vi "InnerCallbackOnWriteTree.vi"(8 "error in":errorcluster, 10 "node (for type)":refnum<class "Engine Parent Editor Node.lvclass">, 11 "node reference":refnum<data-value>) -> (0 "error out":errorcluster)   [LabVIEW 2013, in "PL Framework Configuration Tool.lvlib" / "Engine Parent Editor Node.lvclass"]
uses:
  Engine Parent Editor Node.lvclass
  <vilib>/NI/Configuration Framework/Node/NISE_CEF_Node.lvclass
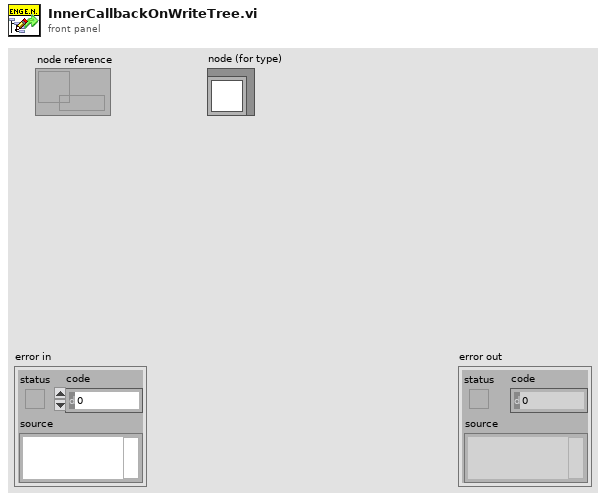
[diagram p1: front panel]
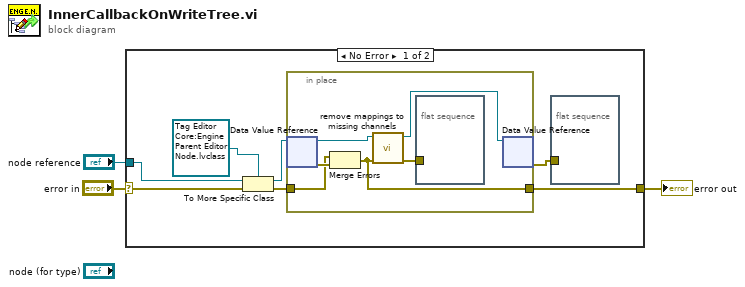
[diagram p0: block diagram]
diagram:
  n1 = case shown="No Error" "error in" {
    selector: "error in" -> [w5 w17]
    tunnel: [w10 w17] -> w3
    tunnel: "node reference" -> [w8 _]
    frame No Error {
      n2 = To More Specific Class(target class=refnum<data-value> refnum, reference=w8, error in=w5) -> (specific class reference=w7:refnum<data-value>, error out=w6:errorcluster)
      n3 = in-place {
        in-place-border: [w12] -> w10
        in-place-border: w6 -> [w11]
        n4 = in-place-dvr #1(w7) -> (w14:refnum<class "Engine Parent Editor Node.lvclass">, w16:errorcluster)
        n5 = Merge Errors(w11, w16) -> (w12:errorcluster)
        n6 = call "remove mappings to missing channels.vi"("error in"=w12, "Engine Parent Editor Node in"=w14) -> ("error out"=w13:errorcluster, "Engine Parent Editor Node out"=w15:refnum<class "Engine Parent Editor Node.lvclass">)  [unwired: 8 in]
        n7 = flat-sequence {
          tunnel: w13 -> [_]
          frame #0 {
          }
        }
        n8 = in-place-dvr #1(w15) -> (w9:errorcluster)  [unwired: 1 out]
      }
      n9 = flat-sequence {
        tunnel: w9 -> [_]
        frame #0 {
        }
      }
    }
    frame Error {
    }
  }
  "error out" <- w3
